vi "HotorNot.vi"() -> ()   [LabVIEW 2013]
panel:
  out "Hot":bool
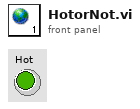
[diagram p1: front panel]
diagram:
